vi "OutputShooter.vi"() -> ()   [LabVIEW 2019]
doc: "This VI runs feedback and feedforward control loops, manages safety interlocks, and sends commands to actuators specific to the shooter subsystem."
uses:
  refnums.vi
  sensors.vi
  outputs.vi
  <vilib>/Rock Robotics/WPI/Solenoid/WPI_SolenoidValue.ctl
  GRNF_GenericMotor.vi
  TAI_Motor.vi
  27d7b9d2-eeda-4251-a250-0f206ebe3d42.vi
  b6d1231e-172b-4004-a400-1c444993ac48.vi
  <vilib>/Rock Robotics/WPI/ThirdParty/Phoenix-LabVIEW/Motor Controller/Controls/CTRE_Phoenix_MotorControl_ControlMode.ctl
  <vilib>/Rock Robotics/WPI/ThirdParty/Phoenix-LabVIEW/Motor Controller/Controls/CTRE_Phoenix_MotorControl_SupplyCurrentLimitConfiguration.ctl
  GRNF_GenericSolenoid.vi
  <vilib>/Rock Robotics/WPI/Solenoid/WPI_SolenoidSetEnum.vi
  TAI_Solenoid.vi
panel:
  in  "Overridden Kicker Speed Goal (rpm)":dbl
  in  "Manually Override Kicker Speed Goal":bool
  in  "Overridden Shooter Speed Goal (rpm)":dbl
  in  "Manually Override Shooter Speed Goal":bool
  in  "Plot Kicker":bool
  out "Kicker":T1(graph)
  in  "Kicker PID":T2={"P Gain"=0.0001, "I Gain"=1e-07, "D Gain"=0.01, "F Gain"=0.0002, "I Zone"=200.0, "Min Output"=0.0, "Max Output"=1.0} {"Max Output" min=-1.0 max=1.0 step=0.01; "Min Output" min=-1.0 max=1.0 step=0.01; "I Zone" step=0.01; "F Gain" step=0.01; "D Gain" step=0.01; "I Gain" step=0.01; "P Gain" min=0.0 step=0.01}
  out "Shooter 1":T1(graph)
  in  "Plot Shooter":bool
  out "Shooter 0":T1(graph)
  in  "Shooter PID":T3={"P Gain"=0.0027, "I Gain"=0.0, "D Gain"=0.007, "F Gain"=0.00017, "I Zone"=200.0} {"I Zone" step=0.01; "F Gain" step=0.01; "D Gain" step=0.01; "I Gain" step=0.01; "P Gain" min=0.0 step=0.01}
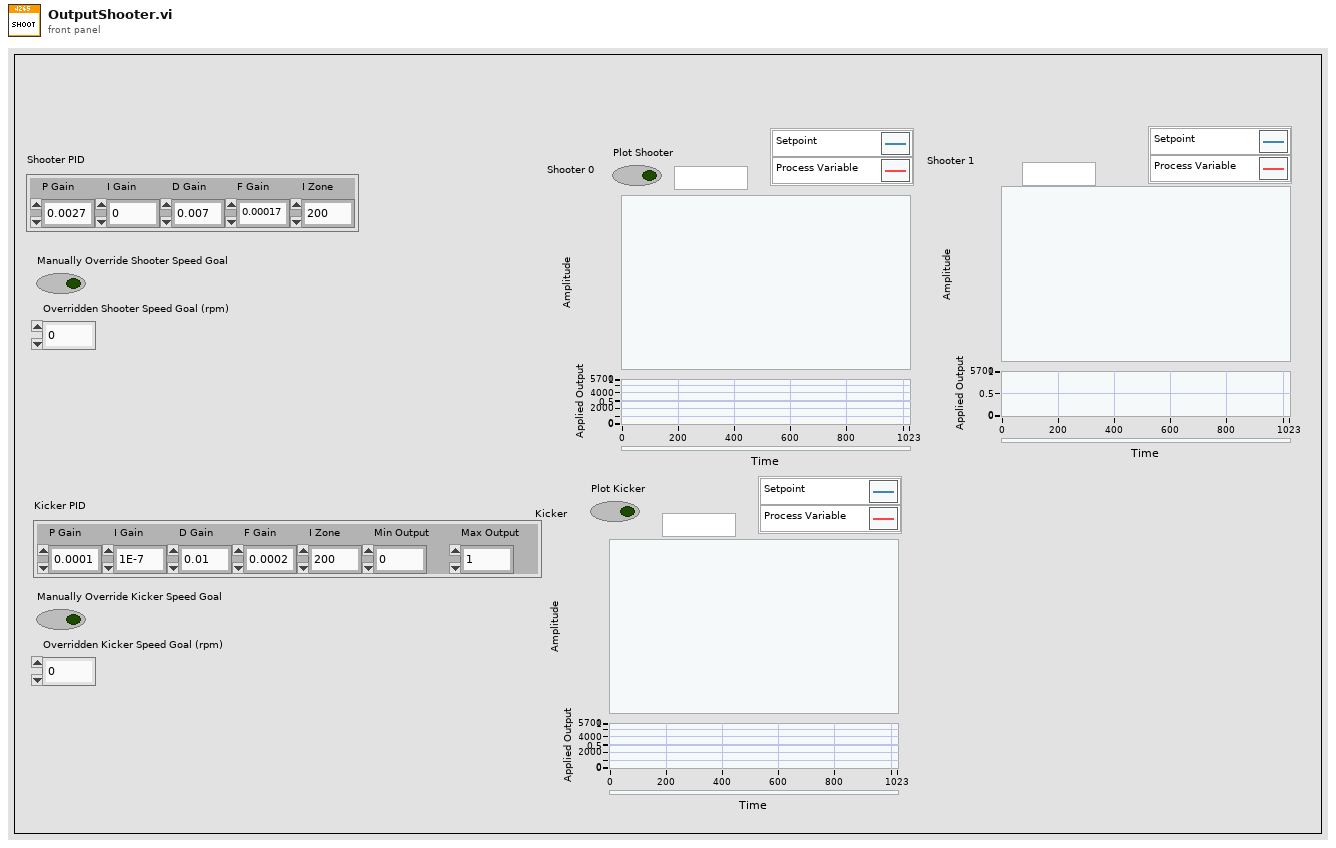
[diagram p1: front panel]
types:
  T1 = cluster{"Sensor Velocity":dbl, "Setpoint":dbl, "Applied Output":dbl}
  T2 = cluster{"P Gain":dbl, "I Gain":dbl, "D Gain":dbl, "F Gain":dbl, "I Zone":dbl, "Min Output":dbl, "Max Output":dbl}
  T3 = cluster{"P Gain":dbl, "I Gain":dbl, "D Gain":dbl, "F Gain":dbl, "I Zone":dbl}
  T4 = typedef "CTRE_Phoenix_MotorControl_ControlMode.ctl" = u16
  T5 = typedef "WPI_MotorControlDeviceRef.ctl" = cluster{"DeviceStatus":errorcluster, "Type":T6, "PWM":cluster{"PWM Channel":T7, "DeadBand":T8}, "CAN":cluster{"Device Number":u8, "SetOutput VI Ref":variant, "GetOutput VI Ref":variant, "Enable VI Ref":variant, "Disable VI Ref":variant, "Data":variant}, "Invert":bool, "DIO PWM":cluster{"PWM \"Enable\" Channel":T7, "DIOChannel":T9, "PWM Rate":dbl}}
  T6 = typedef "WPI_MotorControlType.ctl" = enum16{"PWM", "CAN", "DIO PWM"}
  T7 = typedef "FPGA_DIOPWMChannel.ctl" = enum8{"PWM 0", "PWM 1", "PWM 2", "PWM 3", "PWM 4", "PWM 5", "PWM 6", "PWM 7", "PWM 8", "PWM 9", "PWM MXP 0", "PWM MXP 1", "PWM MXP 2", "PWM MXP 3", "PWM MXP 4", "PWM MXP 5", "PWM MXP 6", "PWM MXP 7", "PWM MXP 8", "PWM MXP 9", "Invalid"}
  T8 = typedef "WPI_PWMDeadband.ctl" = cluster{"Name":string, "maxPositivePwm":i32, "minPositivePwm":i32, "centerPwm":i32, "maxNegativePwm":i32, "minNegativePwm":i32, "angularRange":u16}
  T9 = typedef "FPGA_DIOChannel.ctl" = enum8{"DIO 0", "DIO 1", "DIO 2", "DIO 3", "DIO 4", "DIO 5", "DIO 6", "DIO 7", "DIO 8", "DIO 9", "DIO MXP 0", "DIO MXP 1", "DIO MXP 2", "DIO MXP 3", "DIO MXP 4", "DIO MXP 5", "DIO MXP 6", "DIO MXP 7", "DIO MXP 8", "DIO MXP 9", "DIO MXP 10", "DIO MXP 11", "DIO MXP 12", "DIO MXP 13", "DIO MXP 14", "DIO MXP 15", "SPI Port CS1", "SPI Port CS2", "SPI Port CS3", "SPI Port MISO", "SPI Port MOSI", "Invalid"}
  T10 = typedef "WPI_SolenoidDevRef.ctl" = cluster{"DevStatus":errorcluster, "Pneumatics Control Module":u8, "Forward Solenoid Channel":T11, "Reverse Solenoid Channel":T11}
  T11 = typedef "WPI_SolenoidChannel.ctl" = enum8{"Solenoid 0", "Solenoid 1", "Solenoid 2", "Solenoid 3", "Solenoid 4", "Solenoid 5", "Solenoid 6", "Solenoid 7", "Invalid"}
  T12 = cluster{"P Gain":bool, "I Gain":bool, "D Gain":bool, "F Gain":bool, "I Zone":bool, "Min Output":bool, "Max Output":bool}
  T13 = cluster{"P Gain":bool, "I Gain":bool, "D Gain":bool, "F Gain":bool, "I Zone":bool}
  T14 = typedef "WPI_SolenoidValue.ctl" = enum16{"Off", "On", "Forward", "Reverse"}
  T15 = cluster{"Kicker_Goal_Speed (rpm)***":dbl, "Kicker_Speed (rpm)***":dbl, "Retrieved_Kicker_Power**":dbl}
  T16 = cluster{"Shooter_Goal_Speed (rpm)**":dbl, "Shooter_1_Speed (rpm)**":dbl, "Retrieved_Shooter_1_Power":dbl}
  T17 = cluster{"Shooter_Goal_Speed (rpm)**":dbl, "Shooter_0_Speed (rpm)**":dbl, "Retrieved_Shooter_0_Power":dbl}
  T18 = typedef "CTRE_Phoenix_MotorControl_SupplyCurrentLimitConfiguration.ctl" = cluster{"Enable?":bool, "Current Limit":dbl, "Threshold Current":dbl, "Threshold Time":dbl}
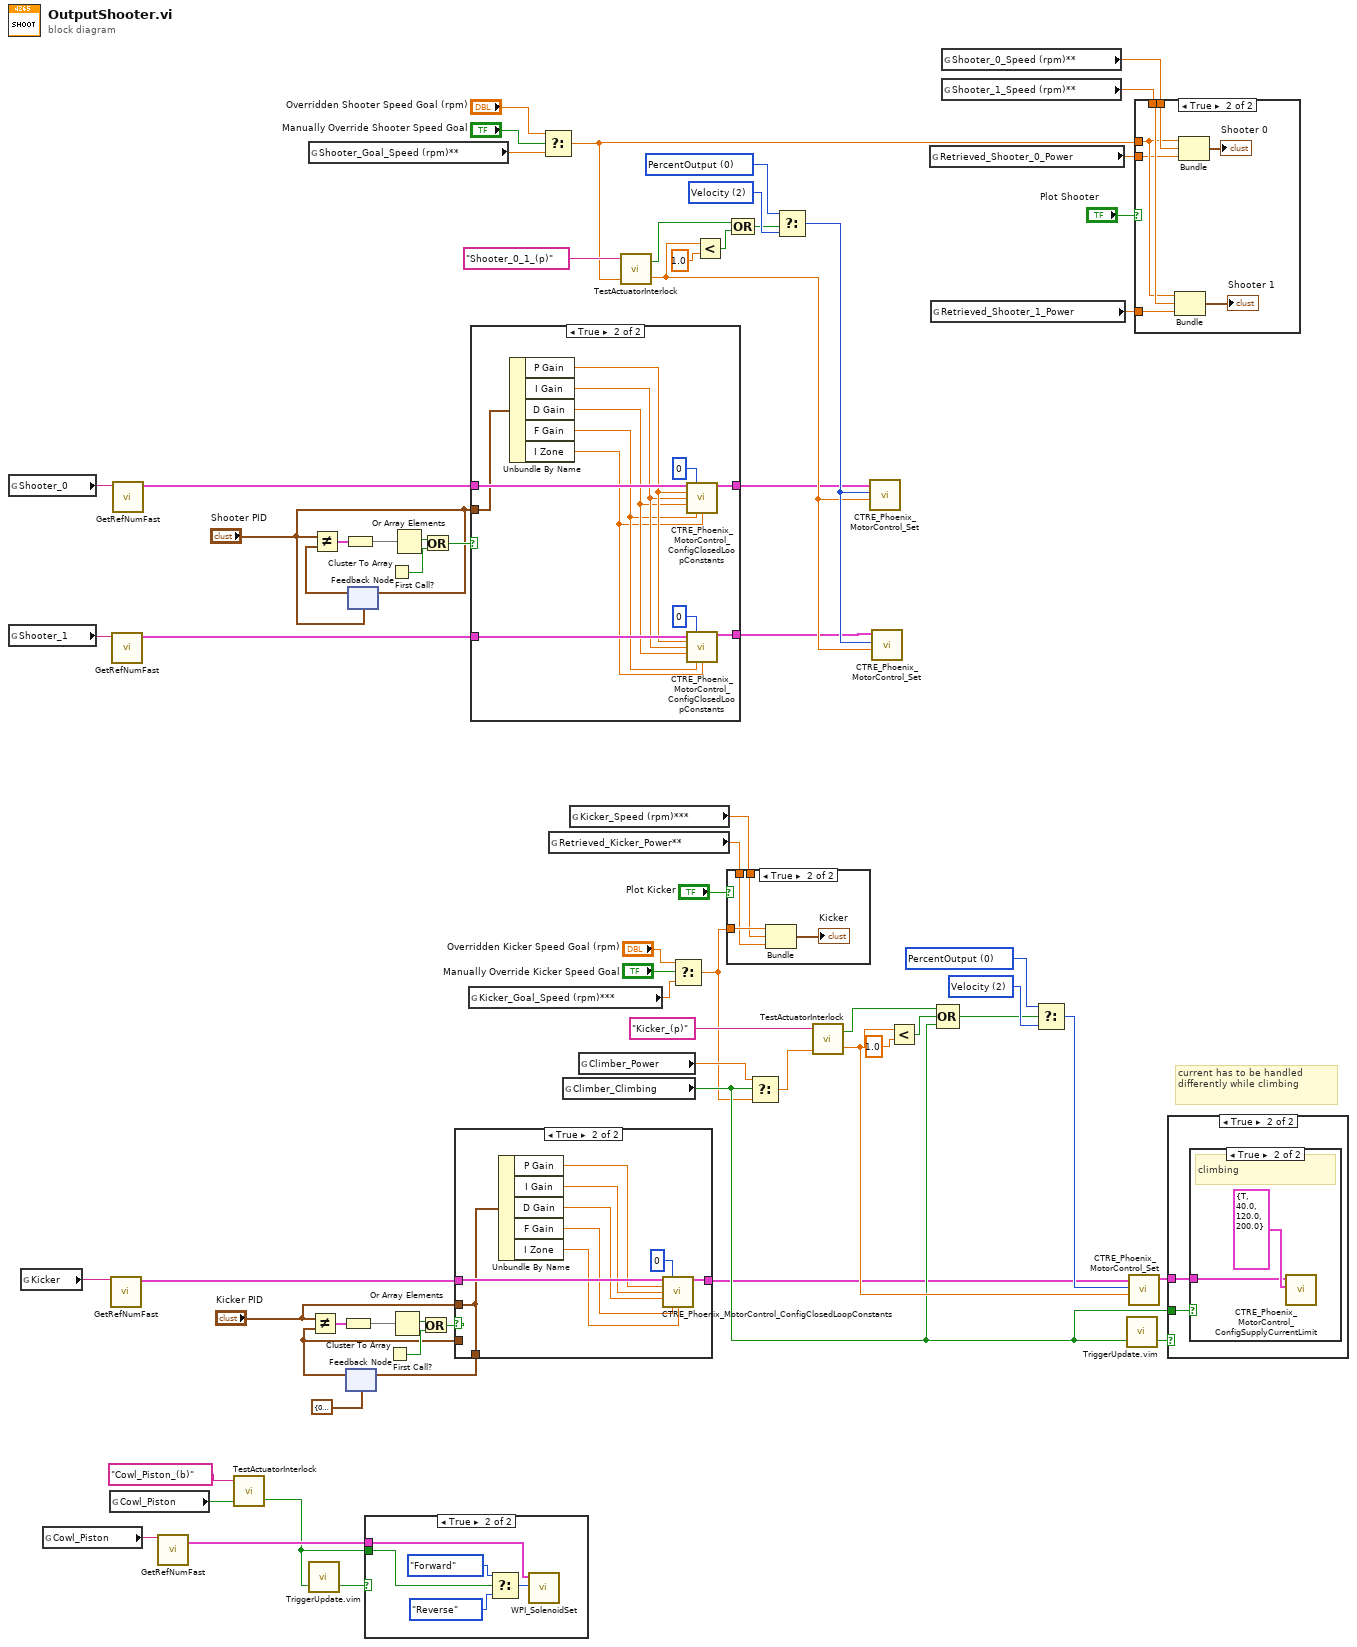
[diagram p0: block diagram]
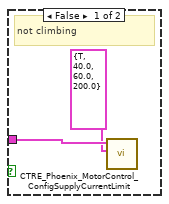
[diagram p4: hidden frame]
diagram:
  w23 = T4 0 items=["PercentOutput"=0, "Position"=1, "Velocity"=2, "Current"=3, "Follower"=5, "MotionProfile"=6, "MotionMagic"=7, "MotionProfileArc"=10, "Disabled"=15] ("Control Mode")
  w22 = T4 2 items=["PercentOutput"=0, "Position"=1, "Velocity"=2, "Current"=3, "Follower"=5, "MotionProfile"=6, "MotionMagic"=7, "MotionProfileArc"=10, "Disabled"=15] ("Control Mode")
  w35 = T4 0 items=["PercentOutput"=0, "Position"=1, "Velocity"=2, "Current"=3, "Follower"=5, "MotionProfile"=6, "MotionMagic"=7, "MotionProfileArc"=10, "Disabled"=15] ("Control Mode")
  w34 = T4 2 items=["PercentOutput"=0, "Position"=1, "Velocity"=2, "Current"=3, "Follower"=5, "MotionProfile"=6, "MotionMagic"=7, "MotionProfileArc"=10, "Disabled"=15] ("Control Mode")
  # "current has to be handled\ndifferently while climbing"
  n1 = global read "refnums.vi" "Shooter_0"() -> (w44:string)
  n2 = global read "refnums.vi" "Shooter_1"() -> (w43:string)
  n3 = global read "refnums.vi" "Kicker"() -> (w42:string)
  n4 = global read "refnums.vi" "Cowl_Piston"() -> (w41:string)
  n5 = global read "outputs.vi" "Cowl_Piston"() -> (w30:bool)
  n6 = call-poly "GetRefNumFast.vi"("RefNum Name"=w42) -> ("Device Reference"=w46:T5)  [unwired: 5 in, 1 out]
  n7 = call-poly "GetRefNumFast.vi"("RefNum Name"=w43) -> ("Device Reference"=w36:T5)  [unwired: 5 in, 1 out]
  n8 = call-poly "GetRefNumFast.vi"("RefNum Name"=w44) -> ("Device Reference"=w47:T5)  [unwired: 5 in, 1 out]
  n9 = call-poly "GetRefNumFast.vi"("RefNum Name"=w41) -> ("Device Reference"=w45:T10)  [unwired: 5 in, 1 out]
  n10 = call-poly "TestActuatorInterlock.vi"("Normal Output"=w30, "Actuator Name"="Cowl_Piston_(b)" ("Actuator_Name")) -> ("Interlock Output"=w31:bool)  [unwired: 1 in, 1 out]
  n11 = global read "outputs.vi" "Shooter_Goal_Speed (rpm)**"() -> (w14:dbl)
  n12 = call "TriggerUpdate.vim"("Trigger"=w31) -> ("Update"=w56:bool)  [unwired: 2 in]
  n13 = feedback #1(T2 {"P Gain"=0.0, "I Gain"=0.0, "D Gain"=0.0, "F Gain"=0.0, "I Zone"=0.0, "Min Output"=0.0, "Max Output"=0.0} ("PID Constants")) -> (w57:T2)
  n14 = Not Equal?(x="Kicker PID", y=w57) -> (x != y?=w61:T12)
  n15 = Cluster To Array(cluster=w61) -> (array=w60:bool[])
  n16 = feedback #2("Shooter PID") -> (w48:T3)
  n17 = Not Equal?(x="Shooter PID", y=w48) -> (x != y?=w50:T13)
  n18 = Cluster To Array(cluster=w50) -> (array=w49:bool[])
  n19 = feedback-in #2("Shooter PID") -> ()
  n20 = case shown="True" w56 {
    tunnel: w31 -> [_ w71]
    tunnel: w45 -> [_ w72]
    frame False {
    }
    frame True {
      n21 = Select(t=WPI_SolenoidValue."Forward" ("Value"), s=w71, f=WPI_SolenoidValue."Reverse" ("Value")) -> (s? t:f=w75:T14)
      n22 = call-poly <vilib>:"WPI_SolenoidSet.vi"("Value"=w75, "SolenoidDevRef"=w72) -> ()  [unwired: 8 in, 2 out]
    }
  }
  n23 = First Call?() -> (First Call?: T/F=w63:bool)
  n24 = First Call?() -> (First Call?: T/F=w52:bool)
  n25 = Or Array Elements(Boolean array=w60) -> (logical OR=w62:bool)
  n26 = Or Array Elements(Boolean array=w49) -> (logical OR=w51:bool)
  n27 = Or(x=w62, y=w63) -> (x .or. y?=w65:bool)
  n28 = Or(x=w51, y=w52) -> (x .or. y?=w53:bool)
  n29 = case shown="True" w65 {
    tunnel: w46 -> [w76 w85]
    tunnel: "Kicker PID" -> [_ w78]
    tunnel: [w77 w78] -> w58
    tunnel: w57 -> [w77 _]
    tunnel: [w76 w86] -> w3
    frame False {
    }
    frame True {
      n30 = Unbundle By Name(w78) -> ("P Gain"=w84:dbl, "I Gain"=w83:dbl, "D Gain"=w82:dbl, "F Gain"=w81:dbl, "I Zone"=w80:dbl)
      n31 = call <vilib>:"CTRE_Phoenix_MotorControl_ConfigClosedLoopConstants.vi"("PhoenixMotorControlDevRef"=w85, "slotIdx"=0, "P"=w84, "I"=w83, "D"=w82, "F"=w81, "I Zone"=w80) -> ("PhoenixMotorControlDevRef"=w86:T5)  [unwired: 7 in, 1 out]
    }
  }
  n32 = feedback-in #1(w58) -> ()
  n33 = global read "outputs.vi" "Kicker_Goal_Speed (rpm)***"() -> (w8:dbl)
  n34 = case shown="True" w53 {
    tunnel: w47 -> [w88 w99]
    tunnel: "Shooter PID" -> [_ w98]
    tunnel: [w88 w100] -> w5
    tunnel: [w87 w97] -> w4
    tunnel: w36 -> [w87 w96]
    frame False {
    }
    frame True {
      n35 = Unbundle By Name(w98) -> ("P Gain"=w95:dbl, "I Gain"=w94:dbl, "D Gain"=w93:dbl, "F Gain"=w92:dbl, "I Zone"=w91:dbl)
      n36 = call <vilib>:"CTRE_Phoenix_MotorControl_ConfigClosedLoopConstants.vi"("PhoenixMotorControlDevRef"=w99, "slotIdx"=0, "P"=w95, "I"=w94, "D"=w93, "F"=w92, "I Zone"=w91) -> ("PhoenixMotorControlDevRef"=w100:T5)  [unwired: 7 in, 1 out]
      n37 = call <vilib>:"CTRE_Phoenix_MotorControl_ConfigClosedLoopConstants.vi"("PhoenixMotorControlDevRef"=w96, "slotIdx"=0, "P"=w95, "I"=w94, "D"=w93, "F"=w92, "I Zone"=w91) -> ("PhoenixMotorControlDevRef"=w97:T5)  [unwired: 7 in, 1 out]
    }
  }
  n38 = Select(t="Overridden Shooter Speed Goal (rpm)", s="Manually Override Shooter Speed Goal", f=w14) -> (s? t:f=w13:dbl)
  n39 = global read "sensors.vi" "Retrieved_Kicker_Power**"() -> (w6:dbl)
  n40 = global read "outputs.vi" "Climber_Climbing"() -> (w15:bool)
  n41 = global read "sensors.vi" "Kicker_Speed (rpm)***"() -> (w67:dbl)
  n42 = global read "outputs.vi" "Climber_Power"() -> (w69:dbl)
  n43 = call-poly "TestActuatorInterlock.vi"("Normal Output"=w13, "Actuator Name"="Shooter_0_1_(p)" ("Actuator_Name")) -> ("Interlock Output"=w28:dbl, "Testing This Actuator"=w26:bool)  [unwired: 1 in]
  n44 = Select(t="Overridden Kicker Speed Goal (rpm)", s="Manually Override Kicker Speed Goal", f=w8) -> (s? t:f=w7:dbl)
  n45 = Less?(x=w28, y=1.0) -> (x < y?=w24:bool)
  n46 = case shown="True" "Plot Kicker" {
    tunnel: w67 -> [_ w103]
    tunnel: w7 -> [_ w104]
    tunnel: w6 -> [_ w101]
    frame False {
    }
    frame True {
      n47 = Bundle("Kicker_Goal_Speed (rpm)***"=w104, "Kicker_Speed (rpm)***"=w103, "Retrieved_Kicker_Power**"=w101) -> (→"Kicker":T15)  [unwired: 1 in]
    }
  }
  n48 = Compound Arithmetic op=OR(w26, w24) -> (w25:bool)
  n49 = Select(t=w69, s=w15, f=w7) -> (s? t:f=w27:dbl)
  n50 = Select(t=w35, s=w25, f=w34) -> (s? t:f=w33:T4)
  n51 = call-poly "TestActuatorInterlock.vi"("Normal Output"=w27, "Actuator Name"="Kicker_(p)" ("Actuator_Name")) -> ("Interlock Output"=w18:dbl, "Testing This Actuator"=w19:bool)  [unwired: 1 in]
  n52 = call <vilib>:"CTRE_Phoenix_MotorControl_Set.vi"("Output"=w28, "Control Mode"=w33, "PhoenixMotorControlDevRef"=w5) -> ()  [unwired: 7 in, 2 out]
  n53 = call <vilib>:"CTRE_Phoenix_MotorControl_Set.vi"("Output"=w28, "Control Mode"=w33, "PhoenixMotorControlDevRef"=w4) -> ()  [unwired: 7 in, 2 out]
  n54 = Less?(x=w18, y=1.0) -> (x < y?=w20:bool)
  n55 = global read "sensors.vi" "Retrieved_Shooter_0_Power"() -> (w2:dbl)
  n56 = global read "sensors.vi" "Retrieved_Shooter_1_Power"() -> (w1:dbl)
  n57 = Compound Arithmetic op=OR(w19, w20, w15) -> (w21:bool)
  n58 = global read "sensors.vi" "Shooter_0_Speed (rpm)**"() -> (w54:dbl)
  n59 = global read "sensors.vi" "Shooter_1_Speed (rpm)**"() -> (w55:dbl)
  n60 = Select(t=w23, s=w21, f=w22) -> (s? t:f=w16:T4)
  n61 = call "TriggerUpdate.vim"("Trigger"=w15) -> ("Update"=w70:bool)  [unwired: 2 in]
  n62 = call <vilib>:"CTRE_Phoenix_MotorControl_Set.vi"("Output"=w18, "Control Mode"=w16, "PhoenixMotorControlDevRef"=w3) -> ("PhoenixMotorControlDevRef"=w29:T5)  [unwired: 7 in, 1 out]
  n63 = case shown="True" "Plot Shooter" {
    tunnel: w55 -> [_ w111]
    tunnel: w54 -> [_ w110]
    tunnel: w13 -> [_ w109]
    tunnel: w2 -> [_ w108]
    tunnel: w1 -> [_ w107]
    frame False {
    }
    frame True {
      n64 = Bundle("Shooter_Goal_Speed (rpm)**"=w109, "Shooter_1_Speed (rpm)**"=w111, "Retrieved_Shooter_1_Power"=w107) -> (→"Shooter 1":T16)  [unwired: 1 in]
      n65 = Bundle("Shooter_Goal_Speed (rpm)**"=w109, "Shooter_0_Speed (rpm)**"=w110, "Retrieved_Shooter_0_Power"=w108) -> (→"Shooter 0":T17)  [unwired: 1 in]
    }
  }
  n66 = case shown="True" w70 {
    tunnel: w29 -> [_ w113]
    tunnel: w15 -> [_ w112]
    frame False {
    }
    frame True {
      n67 = case shown="True" w112 {
        tunnel: w113 -> [w115 w116]
        frame False {
          # "not climbing"
          n68 = call <vilib>:"CTRE_Phoenix_MotorControl_ConfigSupplyCurrentLimit.vi"("Supply Current Limit Configuration"=T18 {"Enable?"=TRUE, "Current Limit"=40.0, "Threshold Current"=60.0, "Threshold Time"=200.0}, "PhoenixMotorControlDevRef"=w115) -> ()  [unwired: 8 in, 2 out]
        }
        frame True {
          # "climbing"
          n69 = call <vilib>:"CTRE_Phoenix_MotorControl_ConfigSupplyCurrentLimit.vi"("Supply Current Limit Configuration"=T18 {"Enable?"=TRUE, "Current Limit"=40.0, "Threshold Current"=120.0, "Threshold Time"=200.0}, "PhoenixMotorControlDevRef"=w116) -> ()  [unwired: 8 in, 2 out]
        }
      }
    }
  }
